vi "Solve Complex Linear Eqs (Gen, multi right hand).vi"(9 "relative tolerance":dbl, 10 "Known Matrix":T1, 11 "Input Matrix":T1) -> (0 "error":i32, 3 "Solution Matrix":T1)   [LabVIEW 2017, in "NI_AALPro.lvlib"]
uses:
  <vilib>/Analysis/NI_AALPro.lvlib
  <vilib>/Analysis/Matrix/Datatypes/ComplexMatrix.ctl
  <resource>/lvanlys.dll
  <vilib>/Analysis/Matrix/NI_Matrix.lvlib
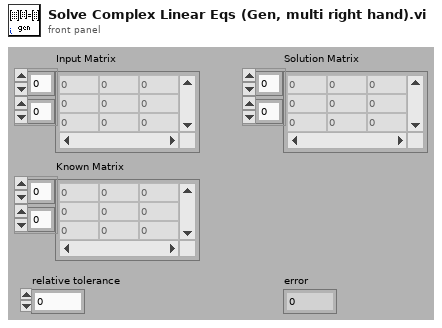
[diagram p1: front panel]
types:
  T1 = typedef "NI_Matrix.lvlib/ComplexMatrix.ctl" = cdb[][]
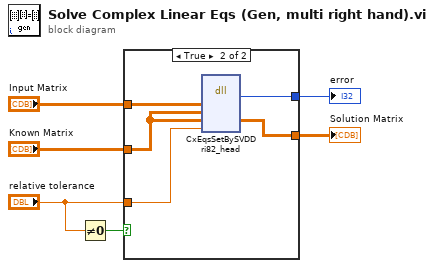
[diagram p0: block diagram]
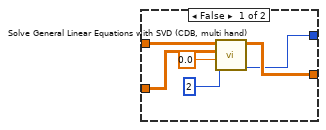
[diagram p2: hidden frame]
diagram:
  n1 = Not Equal To 0?(x="relative tolerance") -> (x != 0?=w6:bool)
  n2 = case shown="True" w6 {
    tunnel: "relative tolerance" -> [_ w15]
    tunnel: "Input Matrix" -> [w12 w17]
    tunnel: "Known Matrix" -> [w11 w16]
    tunnel: [w8 w14] -> w2
    tunnel: [w7 w13] -> w1
    frame False {
      n3 = call <vilib>:"Solve General Linear Equations with SVD (CDB, multi hand).vi"("iteration"=2, "relative tolerance"=0.0, "Known Matrix"=w11, "Input Matrix"=w12) -> ("error"=w7:i32, "Solution Matrix"=w8:T1)  [unwired: 6 in]
    }
    frame True {
      n4 = dll-call lib="e:/builds/penguin/labview/branches/2017/dev/dist/resource/lvanlys.*" fn="CxEqsSetBySVDDri82_head"("aH"=w17, "bH"=w16, "xH"=w16, "relativeTol"=w15) -> ("return type"=w13:i32, "xH"=w14:T1)  [unwired: 6 in, 2 out]
    }
  }
  "Solution Matrix" <- w2
  "error" <- w1
